vi "PrimaryInterfaceGetVariables.vi"(8 "PrimaryInterface":refnum<k24>, 11 "error in":errorcluster) -> (0 "Variables":T1(array[cluster]), 3 "error out":errorcluster)   [LabVIEW 2022 SP3, in "UnderAutomation.UniversalRobots.lvlib"]
uses:
  UnderAutomation.UniversalRobots.lvlib
  C:/Users/fg/Documents/UniversalRobots.vi/LabVIEW_2023/UnderAutomation.UniversalRobots/lib/UnderAutomation.UniversalRobots.dll
  LabVIEW_2023/UnderAutomation.UniversalRobots/lib/UnderAutomation.UniversalRobots.dll
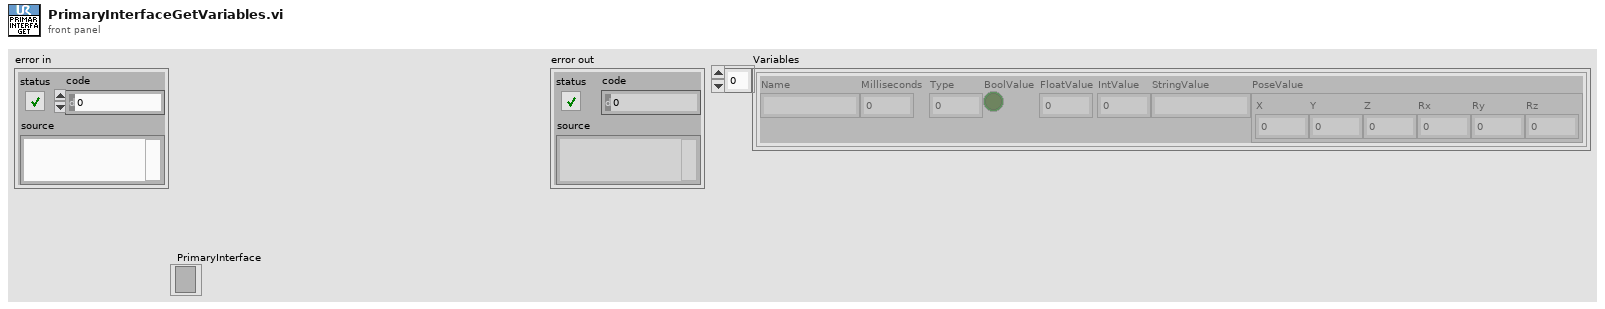
[diagram p1: front panel]
types:
  T1 = cluster{"Name":string, "Milliseconds":i32, "Type":i32, "BoolValue":bool, "FloatValue":sgl, "IntValue":i32, "StringValue":string, "PoseValue":cluster{"X":dbl, "Y":dbl, "Z":dbl, "Rx":dbl, "Ry":dbl, "Rz":dbl}}[]
  T2 = cluster{"Name":string, "Milliseconds":i32, "Type":i32, "BoolValue":bool, "FloatValue":sgl, "IntValue":i32, "StringValue":string, "PoseValue":cluster{"X":dbl, "Y":dbl, "Z":dbl, "Rx":dbl, "Ry":dbl, "Rz":dbl}}
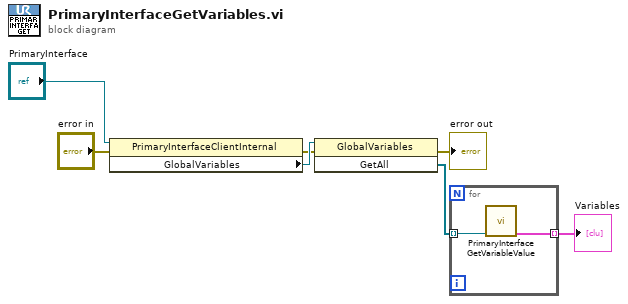
[diagram p0: block diagram]
diagram:
  n1 = property class="PrimaryInterfaceClientInternal"(reference="PrimaryInterface", error in="error in") -> (error out=w2:errorcluster, "GlobalVariables"=w6:refnum<k24>)  [unwired: 1 out]
  n2 = invoke class="GlobalVariables" method="GetAll"(reference=w6, error in=w2) -> (error out=→"error out":errorcluster, "GetAll"=w5:refnum<k24>[])  [unwired: 1 in, 1 out]
  n3 = for {
    tunnel: w5 -> [w9] mode=indexing
    tunnel: [w8] -> w4 mode=indexing
    n4 = call "PrimaryInterfaceGetVariableValue.vi"("Variable"=w9) -> ("Value"=w8:T2)  [unwired: 9 in, 1 out]
  }
  "Variables" <- w4
